vi "niRFUtil WFM Replace Pt by Pt (real array).vi"(0 "Real Array In":T1 min=0 max=127 format="%.2f", 1 "Replace Index":i32, 2 "Replace With":T1 min=0 max=127 format="%.2f", 3 "Default Value (0)":sgl=-inf min=0 max=127 format="%.2f") -> (5 "Real Array Out":T1 min=0 max=127 format="%.2f")   [LabVIEW 2015, in "niRFUtil.lvlib"]
uses:
  niRFUtil.lvlib
  Includes/niRFUtil INC Real Array.ctl
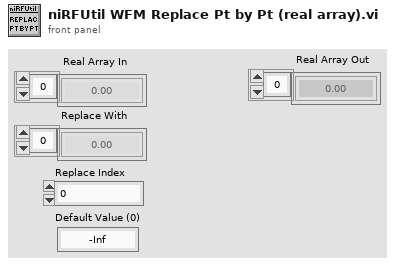
[diagram p1: front panel]
types:
  T1 = typedef "niRFUtil.lvlib/niRFUtil INC Real Array.ctl" = sgl[]
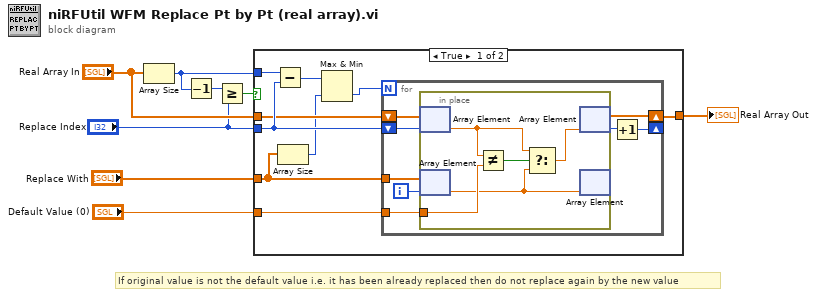
[diagram p0: block diagram]
diagram:
  # "If original value is not the default value i.e. it has been already replaced then do not replace again by the new value"
  n1 = Array Size(array="Real Array In") -> (size(s)=w6:i32)
  n2 = Decrement(x=w6) -> (x-1=w7:i32)
  n3 = Greater Or Equal?(x=w7, y="Replace Index") -> (x >= y?=w8:bool)
  n4 = case shown="True" w8 {
    tunnel: "Real Array In" -> [w16 w31]
    tunnel: [w10 w31] -> w2
    tunnel: "Replace With" -> [w14 _]
    tunnel: "Replace Index" -> [w17 _]
    tunnel: w6 -> [w15 _]
    tunnel: "Default Value (0)" -> [w9 _]
    frame True {
      n5 = Subtract(x=w15, y=w17) -> (x-y=w13:i32)
      n6 = Array Size(array=w14) -> (size(s)=w12:i32)
      n7 = Max & Min(x=w13, y=w12) -> (min(x,y)=w11:i32)  [unwired: 1 out]
      n8 = for {
        N: w11 -> [_]
        shift-right: [w19] -> _
        shift-left: w17 -> [w24]
        shift-right: [w20] -> w10
        shift-left: w16 -> [w25]
        tunnel: w14 -> [w23]
        tunnel: w9 -> [w18]
        i -> [w22]
        n9 = in-place {
          in-place-border: w18 -> [w28]
          n10 = in-place-array #1(w25, w24) -> (w27:sgl)
          n11 = in-place-array #2(w23, w22) -> (w26:sgl)
          n12 = Not Equal?(x=w27, y=w28) -> (x != y?=w30:bool)
          n13 = Select(t=w27, s=w30, f=w26) -> (s? t:f=w29:sgl)
          n14 = in-place-array #1(w29) -> (w20:T1, w21:i32)
          n15 = in-place-array #2(w26) -> ()  [unwired: 2 out]
        }
        n16 = Increment(x=w21) -> (x+1=w19:i32)
      }
    }
    frame False {
    }
  }
  "Real Array Out" <- w2
